vi "Windows Main.vi"() -> ()   [LabVIEW 2016]
panel:
  in  "终端IP地址":string
  out "error out":errorcluster
  in  "停止应用程序":bool
  out "data out":u32[](array[numeric])
  out "Image":T1(plugin-control)
  out "output array":u32[][](array[numeric])
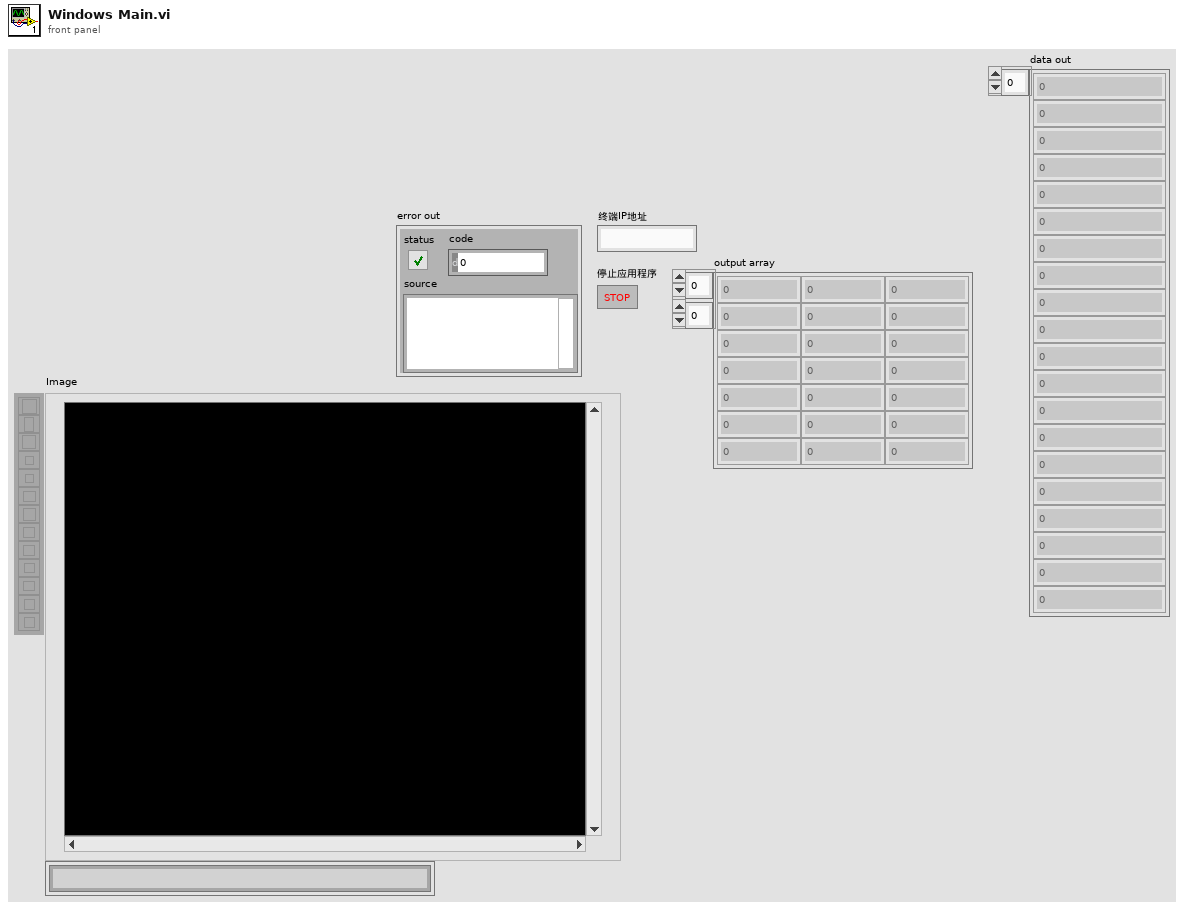
[diagram p1: front panel]
types:
  T1 = typedef "IMAQ Image.ctl" = refnum<image>
  T2 = typedef "Image Type" = u32
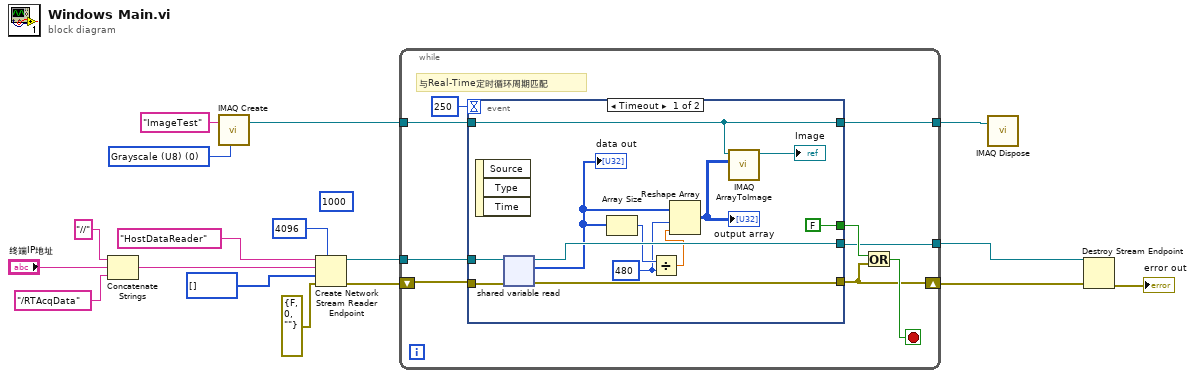
[diagram p0: block diagram]
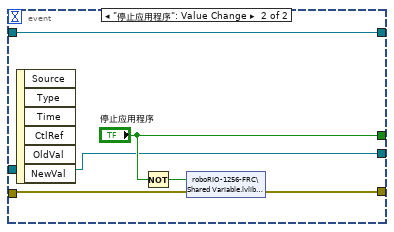
[diagram p2: hidden frame]
diagram:
  w3 = T2 0 items=["Grayscale (U8)", "Grayscale (I16)", "Grayscale (SGL)", "Complex (CSG)", "RGB (U32)", "HSL (U32)", "RGB (U64)", "Grayscale (U16)"] ("Image Type")
  (unwired) 1000 ("timeout in ms (-1)")
  n1 = Concatenate Strings("//" ("string"), "终端IP地址", "/RTAcqData" ("string")) -> (w10:string)
  n2 = call "IMAQ Create"("Image Name"="ImageTest", "Image Type"=w3) -> ("New Image"=w2:T1)  [unwired: 3 in, 1 out]
  n3 = Create Network Stream Reader Endpoint(7:4096 ("reader buffer size"), 8:errorcluster {"status"=FALSE, "code"=0, "source"=""} ("error in (no error)"), 9:i32[] [], 10:w10, 11:"HostDataReader" ("reader name")) -> (0:w17:errorcluster, 3:w8:refnum<k21>)  [unwired: 2 in]
  n4 = while {
    shift-right: [w22] -> w9
    shift-left: w17 -> [w23]
    tunnel: w8 -> [w21]
    tunnel: [w20] -> w7
    tunnel: w2 -> [w19]
    tunnel: [w18] -> w1
    stop <- w24 stop-if-true
    # "与Real-Time定时循环周期匹配"
    n5 = event shown="[0] Timeout" {
      selector: _ -> [_ _]
      dyn-events: _ -> [_ _]
      timeout: 250 -> [_ _]
      tunnel: [FALSE ("停止应用程序") "停止应用程序"] -> w25
      tunnel: w23 -> [w38 w42]
      tunnel: [w37 w41] -> w22
      tunnel: w21 -> [w36 w39]
      tunnel: [w35 w39] -> w20
      tunnel: w19 -> [w27 w40]
      tunnel: [w27 w40] -> w18
      event Timeout {
        w32 = 480 ("y")
        n6 = event-data() -> ()  [unwired: 1 in, 3 out]
        n7 = shared-variable-read(w36, w38) -> (w35:refnum<k21>, w37:errorcluster, w30:i32[])  [unwired: 1 in, 1 out]
        "data out" <- w30
        n8 = Array Size(array=w30) -> (size(s)=w33:i32)
        n9 = Divide(x=w33, y=w32) -> (x/y=w31:dbl)
        n10 = Reshape Array(w30, w32, w31) -> (w29:i32[][])
        "output array" <- w29
        n11 = call "IMAQ ArrayToImage"("Image Pixels (U8)"=w29, "Image"=w27) -> ("Image Out"=→"Image":T1)  [unwired: 8 in, 1 out]
      }
      event "停止应用程序": Value Change {
        n12 = event-data() -> ()  [unwired: 1 in, 6 out]
        n13 = Not(x="停止应用程序") -> (.not. x?=w43:bool)
        n14 = shared-variable "roboRIO-1256-FRC\\Shared Variable.lvlib\\Active"(w43, error in=w42) -> (error out=w41:errorcluster)
      }
    }
    n15 = Or(x=w25, y=w22) -> (x .or. y?=w24:bool)
  }
  n16 = call "IMAQ Dispose"("Image"=w1) -> ()  [unwired: 5 in, 1 out]
  n17 = Destroy Stream Endpoint(8:w9, 11:w7) -> (0:→"error out":errorcluster)
